vi "Configure Digital Threshold.vi"(7 "user value (0.0 V)":dbl caption="User Value (0.0 V)" format="%^.2e", 8 "error in (no error)":errorcluster {"code" format="%.0x"}, 9 "Threshold (TTL)":string(combo)="TTL", 10 "Digital Channel (\"D0\")":string(combo)="DIG0", 11 "VISA Resource Name":refnum<visa-resource-name>) -> (0 "error out":errorcluster {"code" format="%.0x"}, 3 "VISA Resource Name Out":refnum<visa-resource-name>)   [LabVIEW 2011, in "Agilent 546XX Series.lvlib"]
doc: "This VI sets the logical threshold value for all the digital channels grouped with the specified channel (D0-D7, D8-D15). The threshold is used for triggering purposes and for setting the digital data as high (above the threshold) or low (below the threshold).\n\nNOTES: \n\n(1) This VI is only supported by AG546xx\"D\" models. \n\n(2) This VI is only valid for digital channels.\n\n(3) Configuring a digital channel will also configure all the digital channels in the same POD group to the same value."
uses:
  Agilent 546XX Series.lvlib
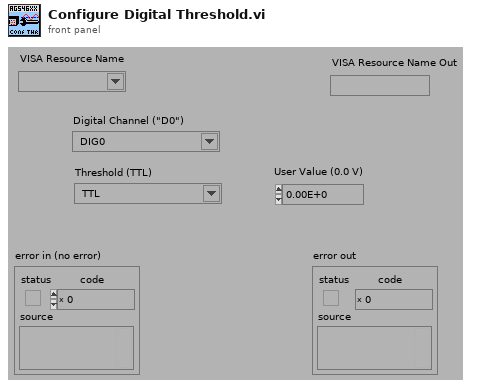
[diagram p1: front panel]
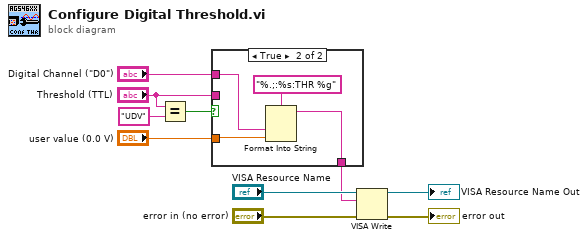
[diagram p0: block diagram]
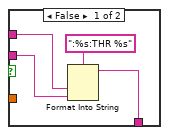
[diagram p2: hidden frame]
diagram:
  n1 = Equal?(x="Threshold (TTL)", y="UDV") -> (x = y?=w5:bool)
  n2 = case shown="True" w5 {
    tunnel: "Digital Channel (\"D0\")" -> [w13 w17]
    tunnel: "Threshold (TTL)" -> [w12 _]
    tunnel: "user value (0.0 V)" -> [_ w18]
    tunnel: [w11 w16] -> w1
    frame False {
      n3 = Format Into String(format string=":%s:THR %s", w13, w12) -> (resulting string=w11:string)  [unwired: 2 in, 1 out]
    }
    frame True {
      n4 = Format Into String(format string="%.;:%s:THR %g", w17, w18) -> (resulting string=w16:string)  [unwired: 2 in, 1 out]
    }
  }
  n5 = VISA Write(VISA resource name="VISA Resource Name", write buffer=w1, error in (no error)="error in (no error)") -> (VISA resource name out=→"VISA Resource Name Out":refnum<visa-resource-name>, error out=→"error out":errorcluster)  [unwired: 1 out]
